vi "DataPacker_SetMIDASPort.vi"(8 "error in (no error)":errorcluster, 10 "Port To Log To":u32, 11 "DataPacker in":refnum<class "DataPacker.lvclass">) -> (0 "error out":errorcluster, 3 "DataPacker out":refnum<class "DataPacker.lvclass">)   [LabVIEW 2018, in "feGEM DataPacker.lvlib" / "DataPacker.lvclass"]
uses:
  DataPacker.lvclass
  DataPacker.lvclass/DataPacker.ctl
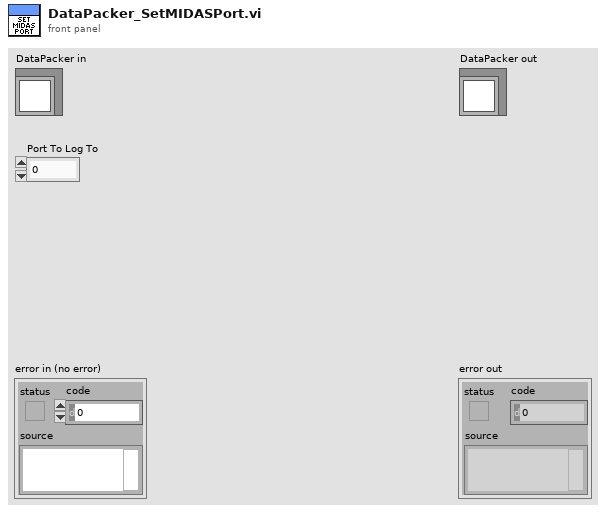
[diagram p1: front panel]
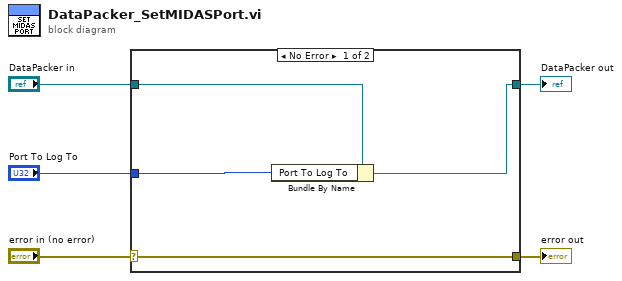
[diagram p0: block diagram]
diagram:
  n1 = case shown="No Error" "error in (no error)" {
    selector: "error in (no error)" -> [w9 w10]
    tunnel: [w9 w10] -> w4
    tunnel: [w7 w11] -> w2
    tunnel: "DataPacker in" -> [w8 w11]
    tunnel: "Port To Log To" -> [w6 _]
    frame No Error {
      n2 = Bundle By Name(cluster=w8, "Port To Log To"=w6) -> (w7:refnum<class "DataPacker.lvclass">)
    }
    frame Error {
    }
  }
  "error out" <- w4
  "DataPacker out" <- w2
